vi "Test Get Summary of Method not Executed .vi"(8 "error in (no error)":errorcluster, 11 "Result Model Result Recording Test in":refnum<class "Result Model Result Recording Test.lvclass">) -> (0 "error out":errorcluster, 3 "Result Model Result Recording Test out":refnum<class "Result Model Result Recording Test.lvclass">)   [LabVIEW 2020, in "Result Model Result Recording Test.lvclass"]
uses:
  Result Model Result Recording Test.lvclass
  source/User Interface/Result Model/Result Model.lvclass
  865a11a4-746d-41de-93c1-4db6b0010296.vi
panel:
  out "Summary":string
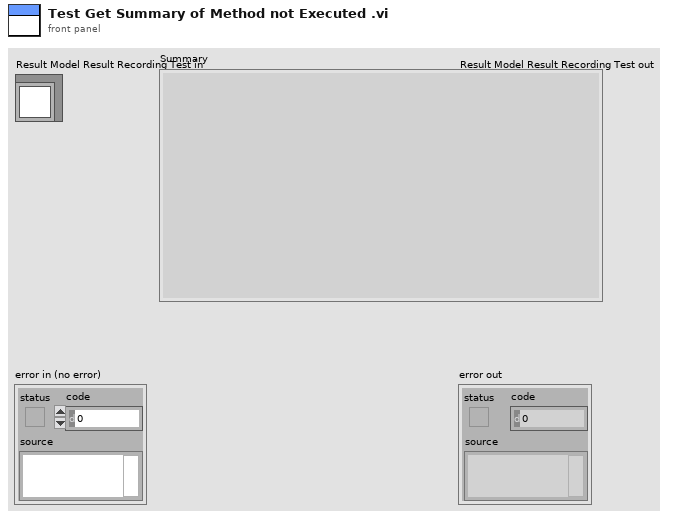
[diagram p1: front panel]
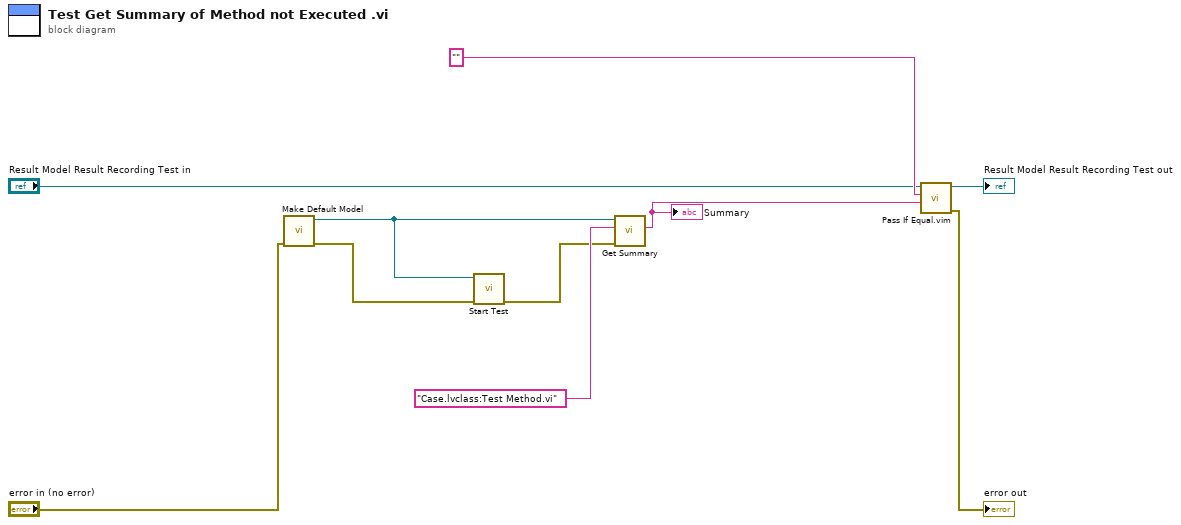
[diagram p0: block diagram]
diagram:
  n1 = call "Make Default Model.vi"("error in (no error)"="error in (no error)") -> ("error out"=w3:errorcluster, "Result Model out"=w1:refnum<class "Result Model.lvclass">)  [unwired: 9 in]
  n2 = call "Start Test.vi"("error in (no error)"=w3, "Result Model by Reference In"=w1) -> ("error out"=w2:errorcluster)  [unwired: 9 in]
  n3 = call "Get Summary.vi"("error in (no error)"=w2, "Item"="Case.lvclass:Test Method.vi", "Result Model by Reference In"=w1) -> ("Summary"=w6:string)  [unwired: 7 in, 1 out]
  "Summary" <- w6
  n4 = call "Pass If Equal.vim"("Actual"=w6, "Expected"="", "LUnit Test Case In"="Result Model Result Recording Test in") -> ("error out"=→"error out":errorcluster, "LUnit Test Case Out"=→"Result Model Result Recording Test out":refnum<class "Result Model Result Recording Test.lvclass">)  [unwired: 7 in]
